vi "Example - Advanced.vi"() -> ()   [LabVIEW 2011]
uses:
  Taskbar Progress Bar.xctl
panel:
  in  "Taskbar Progress Bar":u64(xcontrol)
  in  "Progress Bar Maximum":u64=100
  in  "Clear":bool
  in  "Initialize":bool
  in  "Error":bool
  in  "Pause":bool
  in  "Start Increment":bool
  out "Progress Bar":u64(slide) scale=0.0..100.0
  # "Taskbar Progress  XControl"
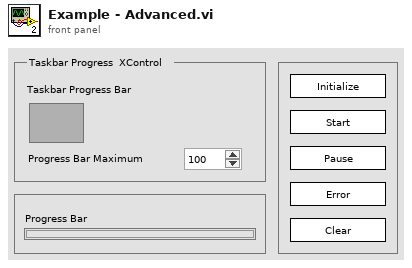
[diagram p1: front panel]
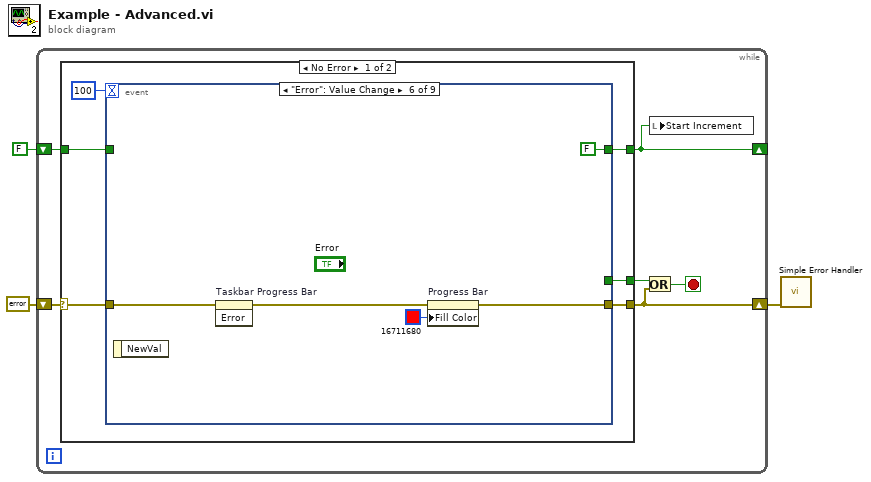
[diagram p0: block diagram]
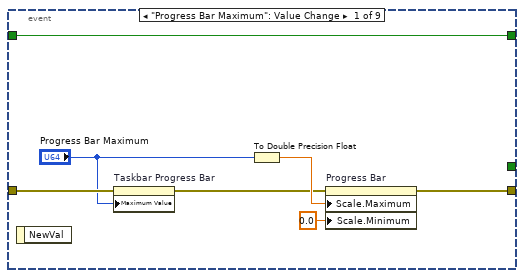
[diagram p2: hidden frame]
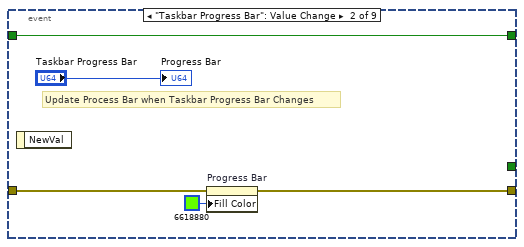
[diagram p3: hidden frame]
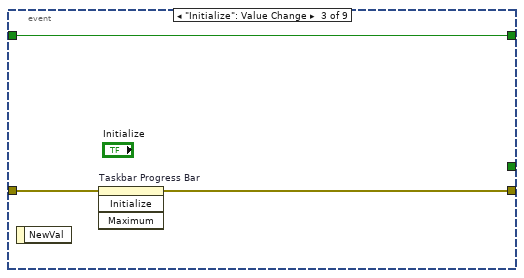
[diagram p4: hidden frame]
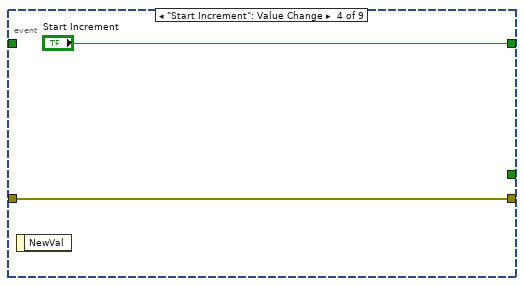
[diagram p5: hidden frame]
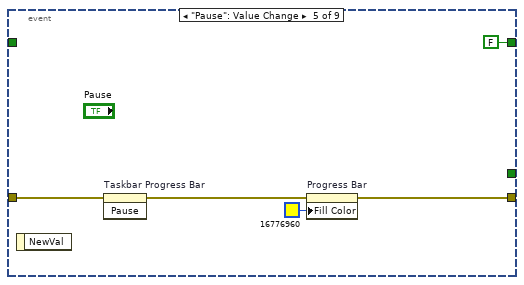
[diagram p6: hidden frame]
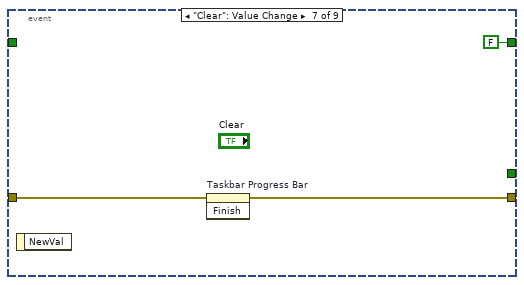
[diagram p7: hidden frame]
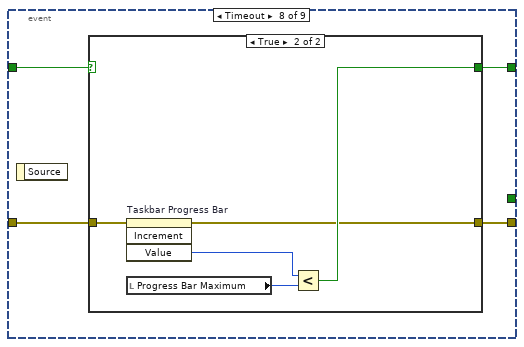
[diagram p8: hidden frame]
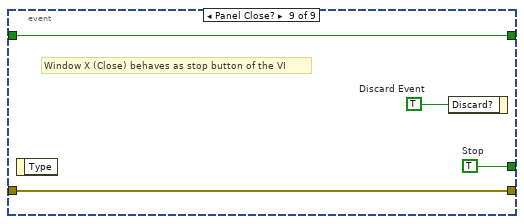
[diagram p10: hidden frame]
diagram:
  n1 = while {
    shift-right: [w6] -> w1
    shift-left: errorcluster {"status"=FALSE, "code"=0, "source"=""} ("error IO") -> [w9]
    shift-right: [w4] -> _
    shift-left: FALSE -> [w5]
    stop <- w7 stop-if-true
    n2 = case shown="No Error" w9 {
      selector: w9 -> [w14 w62]
      tunnel: [w15 _] -> w8
      tunnel: [w13 w62] -> w6
      tunnel: w5 -> [w11 w61]
      tunnel: [w10 w61] -> w4
      frame No Error {
        n3 = event shown="[5] \"Error\": Value Change" {
          selector: _ -> [_ _ _ _ _ _ _ _ _]
          dyn-events: _ -> [_ _ _ _ _ _ _ _ _]
          timeout: 100 -> [_ _ _ _ _ _ _ _ _]
          tunnel: [_ _ _ _ _ _ _ _ w60] -> w15
          tunnel: w14 -> [w18 w25 w29 w32 w34 w39 w43 w49 w59]
          tunnel: [w20 w24 w28 w32 w35 w40 w44 w48 w59] -> w13
          tunnel: w11 -> [w19 w27 w30 _ _ _ _ w47 w57]
          tunnel: [w19 w27 w30 "Start Increment" FALSE FALSE FALSE w46 w57] -> w10
          event "Progress Bar Maximum": Value Change {
            n4 = event-data() -> ()  [unwired: 1 in, 1 out]
            n5 = property on="Taskbar Progress Bar" class="Taskbar Progress Bar (strict)"(error in=w18, "Maximum Value"="Progress Bar Maximum") -> (error out=w17:errorcluster)  [unwired: 1 in, 1 out]
            n6 = To Double Precision Float(number="Progress Bar Maximum") -> (double precision float=w22:dbl)
            n7 = property on="Progress Bar" class="Slide (strict)"(error in=w17, "Scale.Maximum"=w22, "Scale.Minimum"=0.0 ("Scale.Range:Minimum")) -> (error out=w20:errorcluster)  [unwired: 1 in, 1 out]
          }
          event "Taskbar Progress Bar": Value Change {
            # "Update Process Bar when Taskbar Progress Bar Changes"
            n8 = event-data() -> ()  [unwired: 1 in, 1 out]
            n9 = property on="Progress Bar" class="Slide (strict)"(error in=w25, "Fill Color"=u32 6618880) -> (error out=w24:errorcluster)  [unwired: 1 in, 1 out]
            "Progress Bar" <- "Taskbar Progress Bar"
          }
          event "Initialize": Value Change {
            n10 = event-data() -> ()  [unwired: 1 in, 1 out]
            n11 = invoke on="Taskbar Progress Bar" class="Taskbar Progress Bar (strict)" method="Initialize"(error in=w29) -> (error out=w28:errorcluster)  [unwired: 3 in, 3 out]
          }
          event "Start Increment": Value Change {
            n12 = event-data() -> ()  [unwired: 1 in, 1 out]
          }
          event "Pause": Value Change {
            n13 = event-data() -> ()  [unwired: 1 in, 1 out]
            n14 = invoke on="Taskbar Progress Bar" class="Taskbar Progress Bar (strict)" method="Pause"(error in=w34) -> (error out=w33:errorcluster)  [unwired: 2 in, 2 out]
            n15 = property on="Progress Bar" class="Slide (strict)"(error in=w33, "Fill Color"=u32 16776960) -> (error out=w35:errorcluster)  [unwired: 1 in, 1 out]
          }
          event "Error": Value Change {
            n16 = event-data() -> ()  [unwired: 1 in, 1 out]
            n17 = invoke on="Taskbar Progress Bar" class="Taskbar Progress Bar (strict)" method="Error"(error in=w39) -> (error out=w38:errorcluster)  [unwired: 2 in, 2 out]
            n18 = property on="Progress Bar" class="Slide (strict)"(error in=w38, "Fill Color"=u32 16711680) -> (error out=w40:errorcluster)  [unwired: 1 in, 1 out]
          }
          event "Clear": Value Change {
            n19 = event-data() -> ()  [unwired: 1 in, 1 out]
            n20 = invoke on="Taskbar Progress Bar" class="Taskbar Progress Bar (strict)" method="Finish"(error in=w43) -> (error out=w44:errorcluster)  [unwired: 2 in, 2 out]
          }
          event Timeout {
            n21 = event-data() -> ()  [unwired: 1 in, 1 out]
            n22 = case shown="True" w47 {
              selector: w47 -> [w50 _]
              tunnel: w49 -> [w51 w54]
              tunnel: [w51 w53] -> w48
              tunnel: [w50 w55] -> w46
              frame False {
              }
              frame True {
                n23 = invoke on="Taskbar Progress Bar" class="Taskbar Progress Bar (strict)" method="Increment"(error in=w54) -> (error out=w53:errorcluster, "Value"=w52:u64)  [unwired: 3 in, 2 out]
                n24 = local read "Progress Bar Maximum"() -> (w56:u64)
                n25 = Less?(x=w52, y=w56) -> (x < y?=w55:bool)
              }
            }
          }
          event Panel Close? {
            w58 = TRUE  # Discard Event
            w60 = TRUE  # Stop
            # "Window X (Close) behaves as stop button of the VI"
            n26 = event-data() -> ()  [unwired: 1 in, 1 out]
            n27 = event-data("Discard?"=w58) -> ()  [unwired: 1 in, 1 out]
          }
        }
      }
      frame Error {
      }
    }
    n28 = Or(x=w8, y=w6) -> (x .or. y?=w7:bool)
    n29 = local write "Start Increment"(w4) -> ()
  }
  n30 = call <vilib>:"Simple Error Handler.vi"("error in (no error)"=w1) -> ()  [unwired: 4 in, 5 out]
